vi "Exercício 2.vi"() -> ()   [LabVIEW 2016]
panel:
  out "Superior a 40º":bool
  out "30<T<40":bool
  out "Inferior a 30º":bool
  in  "stop":bool
  in  "Resistência":dbl
  out "Temperatura":dbl
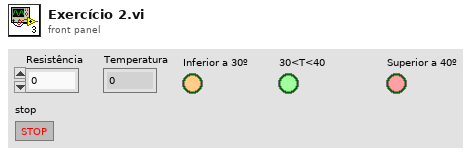
[diagram p1: front panel]
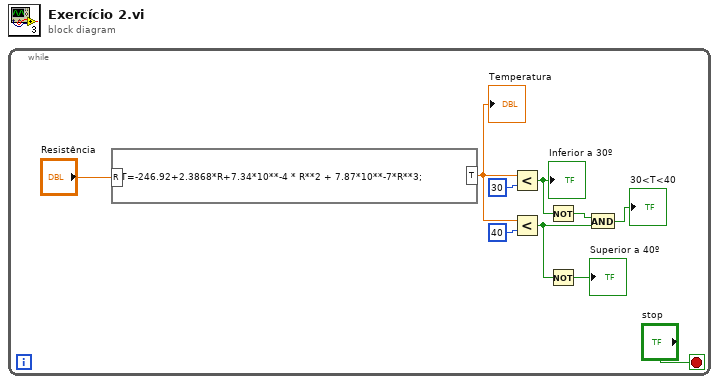
[diagram p0: block diagram]
diagram:
  n1 = while {
    stop <- "stop" stop-if-true
    n2 = formula code="T=-246.92+2.3868*R+7.34*10**-4 * R**2 + 7.87*10**-7*R**3;"("R"="Resistência") -> ("T"=w1:dbl)
    "Temperatura" <- w1
    n3 = Less?(x=w1, y=30) -> (x < y?=w7:bool)
    "Inferior a 30º" <- w7
    n4 = Less?(x=w1, y=40) -> (x < y?=w3:bool)
    n5 = Not(x=w7) -> (.not. x?=w5:bool)
    n6 = Not(x=w3) -> (.not. x?=→"Superior a 40º":bool)
    n7 = And(x=w5, y=w3) -> (x .and. y?=→"30<T<40":bool)
  }
